vi "main.vi"() -> ()   [LabVIEW 2021]
panel:
  in  "VALHTSw":bool
  in  "Stop":bool
  in  "SPVALLT":u8 max=100
  in  "SPVALHT":u8 max=100
  out "DPTSYS":sgl format="%#_3g"
  out "DPTOT":sgl format="%#_2g"
  out "DPVALLT":sgl
  out "DPVALHT":sgl
  out "DPTEGLT":sgl
  out "DPTEGHT":sgl
  out "posVALLT":sgl(knob) scale=0.0..100.0
  out "posVALHT":sgl(knob) scale=0.0..100.0
  out "Boolean":bool
  # "%"
  # "%"
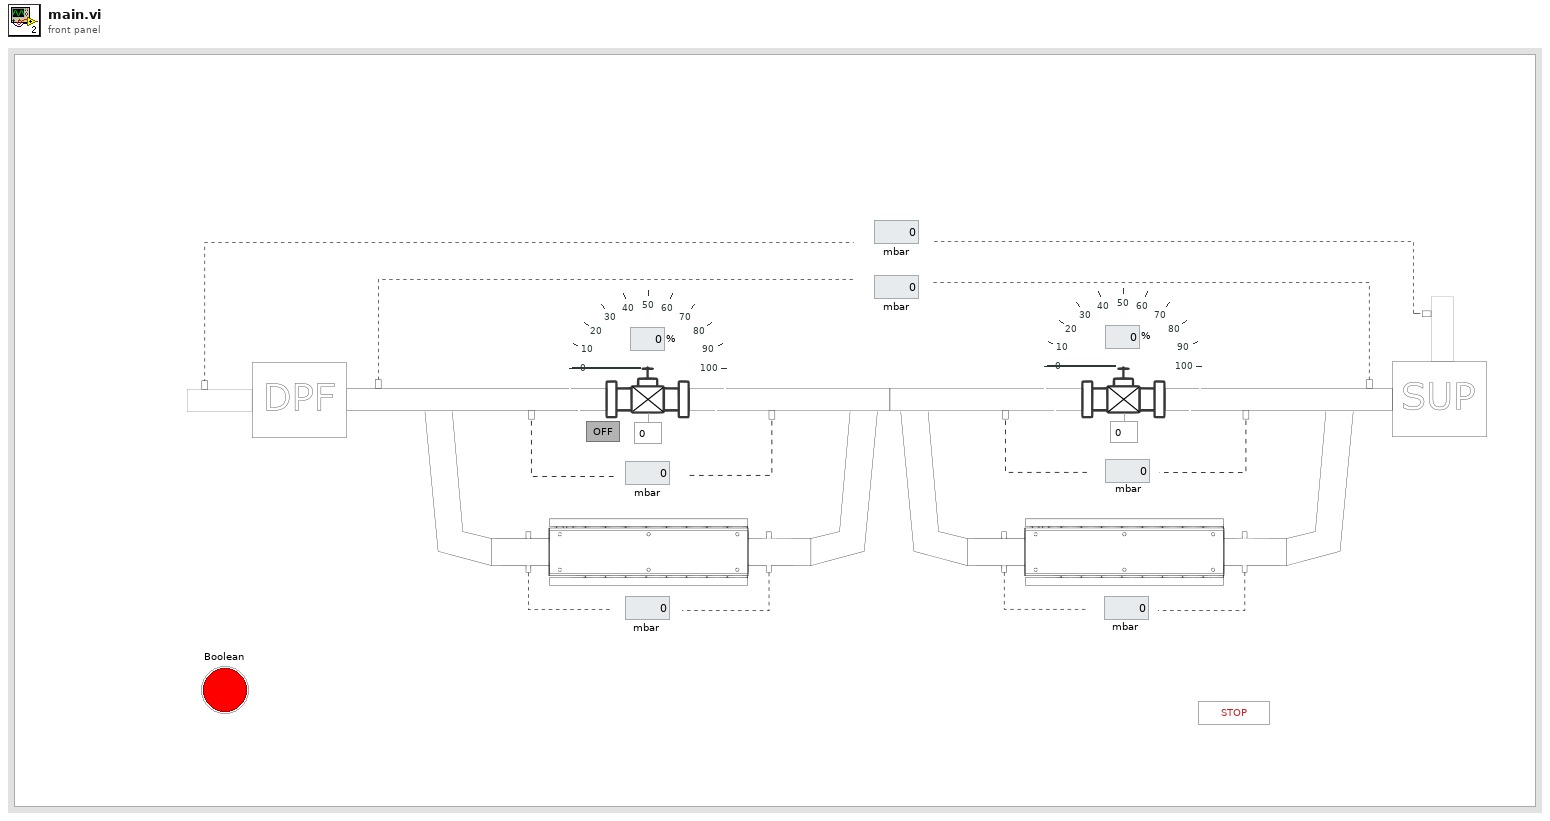
[diagram p1: front panel]
types:
  T1 = cluster{"ValvePos1":sgl, "ValvePos2":sgl, "PressureArray":sgl[], "TempArray2":sgl[], "TempArray1":sgl[]}[]
  T2 = enum16{"waiting", "connect to tcp server", "configuration", "data logging", "saving data and close connection"}
  T3 = enum16{"Disconnected", "Connecting", "Conected", "Sending"}
  T4 = cluster{"ValvePos1":i32, "ValvePos2":i32, "PressureArray":sgl[], "TempArray2":sgl[], "TempArray1":sgl[]}
  T5 = cluster{"ValvePos1":sgl, "ValvePos2":sgl, "PressureArray":sgl[], "TempArray2":sgl[], "TempArray1":sgl[]}
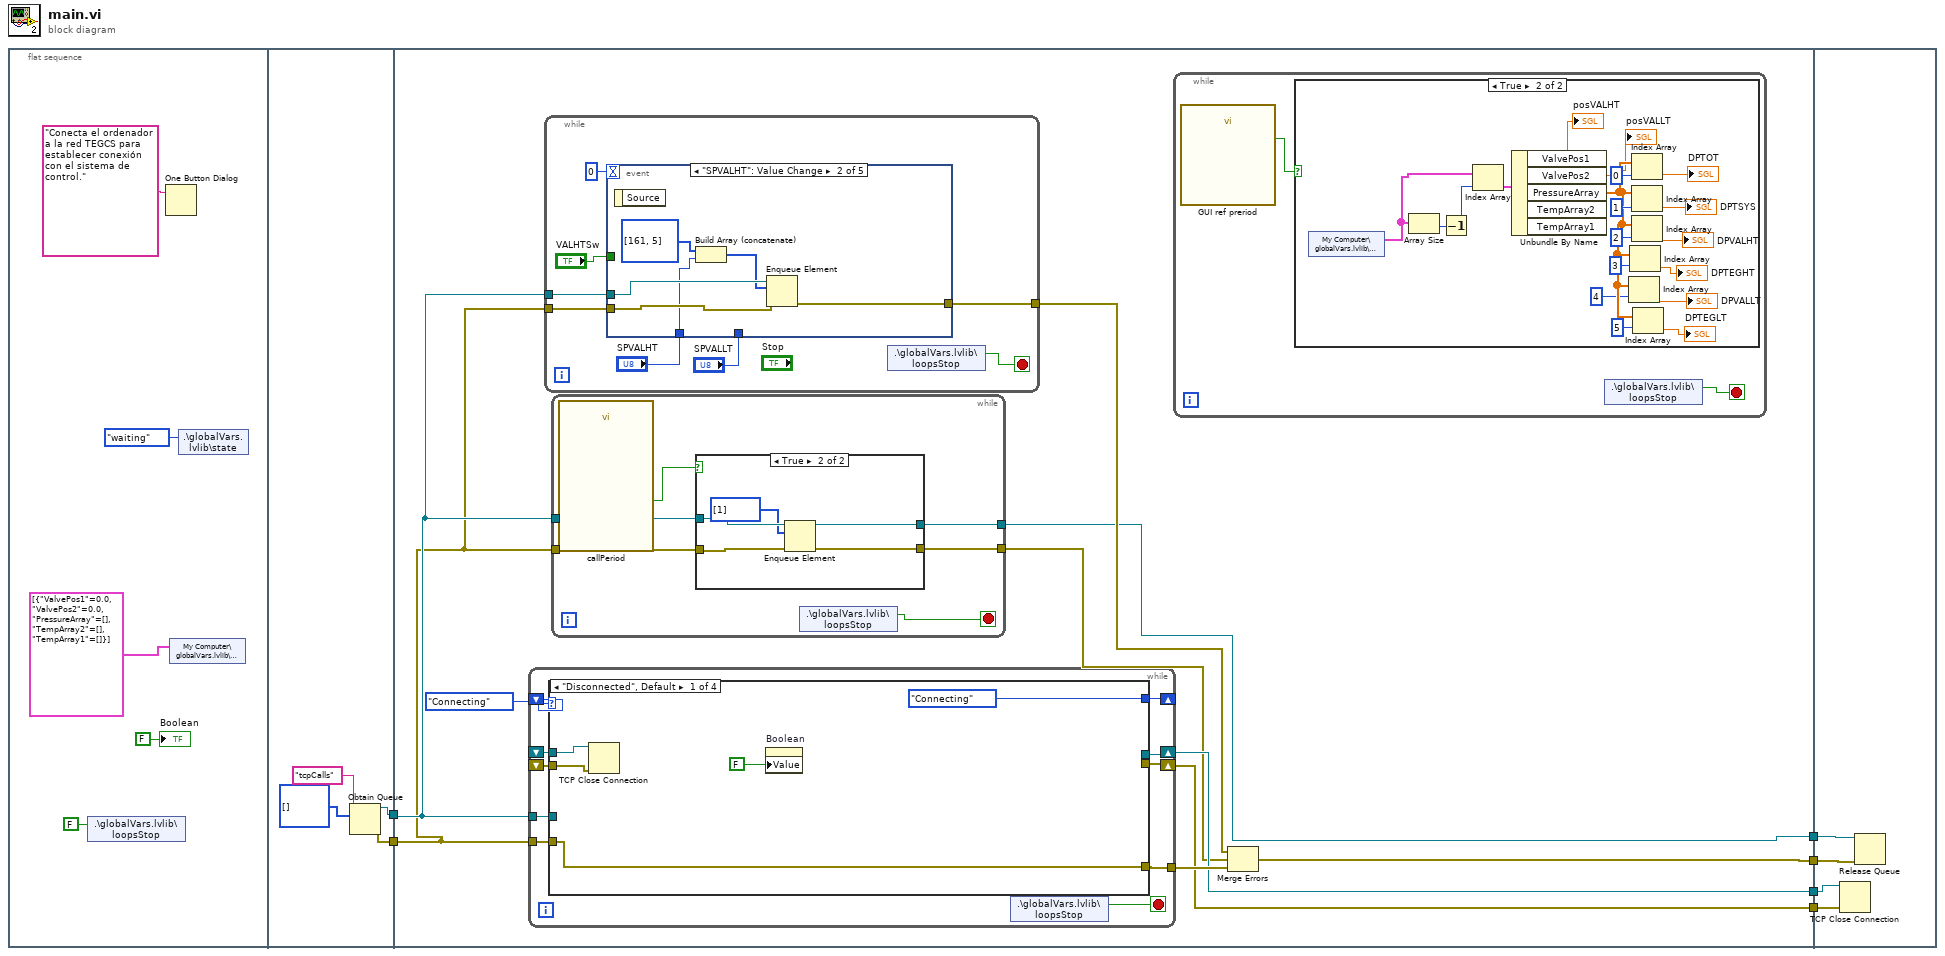
[diagram p0: block diagram]
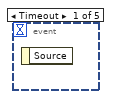
[diagram p2: hidden frame]
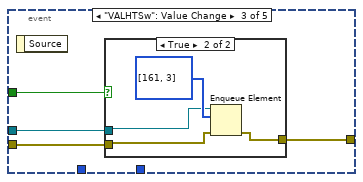
[diagram p3: hidden frame]
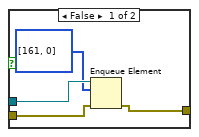
[diagram p4: hidden frame]
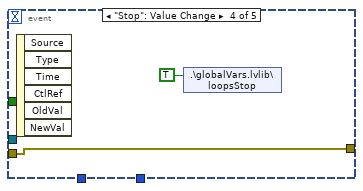
[diagram p5: hidden frame]
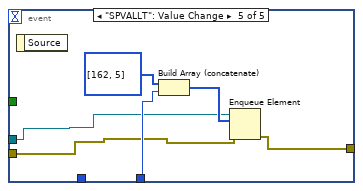
[diagram p6: hidden frame]
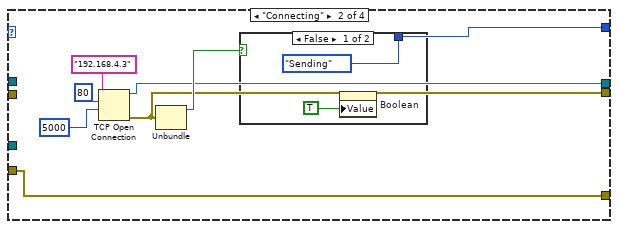
[diagram p9: hidden frame]
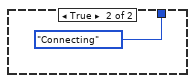
[diagram p10: hidden frame]
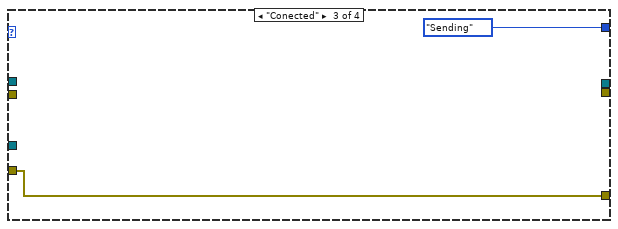
[diagram p11: hidden frame]
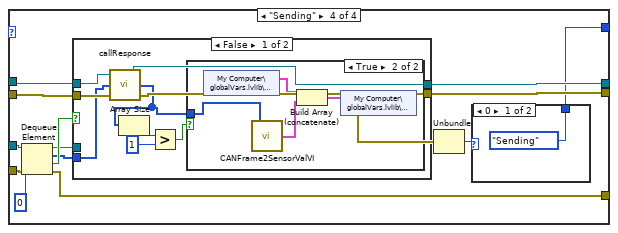
[diagram p12: hidden frame]
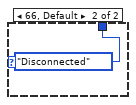
[diagram p13: hidden frame]
diagram:
  n1 = flat-sequence {
    tunnel: [w13] -> w6
    tunnel: [w12] -> w5
    tunnel: w6 -> [w23]
    tunnel: w5 -> [w24]
    tunnel: [w21] -> w4
    tunnel: [w16] -> w3
    tunnel: [w20] -> w2
    tunnel: [w19] -> w1
    tunnel: w4 -> [w155]
    tunnel: w3 -> [w154]
    tunnel: w2 -> [w153]
    tunnel: w1 -> [w152]
    frame #0 {
      n2 = shared-variable ".\\globalVars.lvlib\\loopsStop"(FALSE ("loopsStop")) -> ()  [unwired: 1 in, 1 out]
      n3 = One Button Dialog(message="Conecta el ordenador a la red TEGCS para establecer conexión con el sistema de control.") -> ()  [unwired: 1 in, 1 out]
      n4 = shared-variable "My Computer\\globalVars.lvlib\\sensD"(T1 [{"ValvePos1"=0.0, "ValvePos2"=0.0, "PressureArray"=[], "TempArray2"=[], "TempArray1"=[]}] ("sensD")) -> ()  [unwired: 1 in, 1 out]
      n5 = shared-variable ".\\globalVars.lvlib\\state"(T2."waiting" ("state")) -> ()  [unwired: 1 in, 1 out]
      "Boolean" <- FALSE ("Boolean")
    }
    frame #1 {
      n6 = Obtain Queue(name (unnamed)="tcpCalls", element data type=u8[] [] ("Array")) -> (queue out=w12:refnum<queue>, error out=w13:errorcluster)  [unwired: 3 in, 1 out]
    }
    frame #2 {
      n7 = while {
        shift-right: [w100] -> _
        shift-left: T3."Connecting" -> [w103]
        shift-right: [w102] -> w19
        shift-left: _ -> [w99]
        shift-right: [w101] -> w20
        shift-left: _ -> [w98]
        tunnel: w23 -> [w97]
        tunnel: w24 -> [w96]
        tunnel: [w94] -> w22
        stop <- w95 stop-if-true
        n8 = case shown="\"Disconnected\", Default" w103 {
          tunnel: [T3."Connecting" w113 T3."Sending" w125] -> w100
          tunnel: [_ w111 _ w128] -> w102
          tunnel: [_ w110 _ w127] -> w101
          tunnel: w99 -> [w108 _ _ w130]
          tunnel: w98 -> [w107 _ _ w129]
          tunnel: w97 -> [w104 w109 w120 w133]
          tunnel: w96 -> [_ _ _ w134]
          tunnel: [w104 w109 w120 w124] -> w94
          frame "Disconnected", Default {
            n9 = TCP Close Connection(connection ID=w108, error in (no error)=w107) -> ()  [unwired: 1 in, 2 out]
            n10 = property on="Boolean" class="Bool (strict)"("Value"=FALSE ("Boolean")) -> ()  [unwired: 2 in, 2 out]
          }
          frame "Connecting" {
            n11 = TCP Open Connection(address="192.168.4.3", remote port or service name=u16 80, timeout ms (60000)=5000) -> (connection ID=w111:refnum<k5>, error out=w110:errorcluster)  [unwired: 2 in]
            n12 = Unbundle(w110) -> ("status"=w112:bool)  [unwired: 2 out]
            n13 = case shown="False" w112 {
              tunnel: [T3."Sending" T3."Connecting"] -> w113
              frame False {
                n14 = property on="Boolean" class="Bool (strict)"("Value"=TRUE ("Boolean")) -> ()  [unwired: 2 in, 2 out]
              }
              frame True {
              }
            }
          }
          frame "Conected" {
          }
          frame "Sending" {
            n15 = Dequeue Element(queue=w134, timeout in ms (-1)=0, error in (no error)=w133) -> (queue out=w123:refnum<queue>, element=w122:u8[], timed out?=w131:bool, error out=w124:errorcluster)
            n16 = case shown="False" w131 {
              tunnel: w130 -> [w145 w150]
              tunnel: w129 -> [w144 w151]
              tunnel: [w143 w151] -> w127
              tunnel: [w142 w150] -> w128
              tunnel: w123 -> [_ _]
              tunnel: w122 -> [w141 _]
              frame False {
                n17 = call "callResponse.vi"("error in (no error)"=w144, "input"=w141, "TCP Network Connection in"=w145) -> ("error out"=w143:errorcluster, "unsigned byte array"=w137:u8[], "TCP Network Connection out"=w142:refnum<k5>)
                n18 = Array Size(array=w137) -> (size(s)=w140:i32)
                n19 = Greater?(x=w140, y=1) -> (0:w138:bool)
                n20 = case shown="True" w138 {
                  tunnel: w137 -> [_ w148]
                  frame False {
                  }
                  frame True {
                    n21 = shared-variable "My Computer\\globalVars.lvlib\\sensD"() -> (w146:T1)  [unwired: 1 in, 1 out]
                    n22 = call "CANFrame2SensorValVI.vi"("input"=w148) -> ("output data cluster"=w149:T4)
                    n23 = Build Array (concatenate)(w146, w149) -> (w147:T1)
                    n24 = shared-variable "My Computer\\globalVars.lvlib\\sensD"(w147) -> ()  [unwired: 1 in, 1 out]
                  }
                }
              }
              frame True {
              }
            }
            n25 = Unbundle(w127) -> ("code"=w126:i32)  [unwired: 2 out]
            n26 = case shown="0" w126 {
              tunnel: [T3."Sending" T3."Disconnected"] -> w125
              frame 0 {
              }
              frame 66, Default {
              }
            }
          }
        }
        n27 = shared-variable ".\\globalVars.lvlib\\loopsStop"() -> (w95:bool)  [unwired: 1 in, 1 out]
      }
      n28 = while {
        tunnel: w24 -> [w30]
        tunnel: w23 -> [w32]
        tunnel: [w27] -> w17
        stop <- w29 stop-if-true
        n29 = event shown="[1] \"SPVALHT\": Value Change" {
          selector: _ -> [_ _ _ _ _]
          dyn-events: _ -> [_ _ _ _ _]
          timeout: 0 -> [_ _ _ _ _]
          tunnel: w32 -> [_ w38 w43 w52 w56]
          tunnel: "SPVALHT" -> [_ w36 _ _ _]
          tunnel: w30 -> [_ w39 w42 _ w55]
          tunnel: "SPVALLT" -> [_ _ _ _ w57]
          tunnel: [_ w34 w40 w52 w54] -> w27
          tunnel: "VALHTSw" -> [_ _ w41 _ _]
          event Timeout {
            n30 = event-data() -> ()  [unwired: 1 in, 1 out]
          }
          event "SPVALHT": Value Change {
            n31 = event-data() -> ()  [unwired: 1 in, 1 out]
            n32 = Build Array (concatenate)(u8[] [161, 5] ("element"), w36) -> (w35:u8[])
            n33 = Enqueue Element(queue=w39, element=w35, error in (no error)=w38) -> (error out=w34:errorcluster)  [unwired: 1 in, 2 out]
          }
          event "VALHTSw": Value Change {
            n34 = event-data() -> ()  [unwired: 1 in, 1 out]
            n35 = case shown="True" w41 {
              tunnel: w43 -> [w47 w49]
              tunnel: w42 -> [w46 w50]
              tunnel: [w44 w48] -> w40
              frame False {
                n36 = Enqueue Element(queue=w46, element=u8[] [161, 0], error in (no error)=w47) -> (error out=w44:errorcluster)  [unwired: 1 in, 2 out]
              }
              frame True {
                n37 = Enqueue Element(queue=w50, element=u8[] [161, 3], error in (no error)=w49) -> (error out=w48:errorcluster)  [unwired: 1 in, 2 out]
              }
            }
          }
          event "Stop": Value Change {
            n38 = event-data() -> ()  [unwired: 1 in, 6 out]
            n39 = shared-variable ".\\globalVars.lvlib\\loopsStop"(TRUE ("loopsStop")) -> ()  [unwired: 1 in, 1 out]
          }
          event "SPVALLT": Value Change {
            n40 = event-data() -> ()  [unwired: 1 in, 1 out]
            n41 = Build Array (concatenate)(u8[] [162, 5] ("element"), w57) -> (w58:u8[])
            n42 = Enqueue Element(queue=w55, element=w58, error in (no error)=w56) -> (error out=w54:errorcluster)  [unwired: 1 in, 2 out]
          }
        }
        n43 = shared-variable ".\\globalVars.lvlib\\loopsStop"() -> (w29:bool)  [unwired: 1 in, 1 out]
      }
      n44 = while {
        tunnel: w24 -> [w84]
        tunnel: w23 -> [w85]
        tunnel: [w83] -> w18
        tunnel: [w82] -> w16
        stop <- w81 stop-if-true
        n45 = call "callPeriod"() -> ("Time has Elapsed"=w86:bool)  [unwired: 12 in, 7 out]
        n46 = case shown="True" w86 {
          tunnel: w85 -> [w88 w92]
          tunnel: w84 -> [w87 w93]
          tunnel: [w88 w90] -> w83
          tunnel: [w87 w89] -> w82
          frame False {
          }
          frame True {
            n47 = Enqueue Element(queue=w93, element=u8[] [1], error in (no error)=w92) -> (queue out=w89:refnum<queue>, error out=w90:errorcluster)  [unwired: 1 in, 1 out]
          }
        }
        n48 = shared-variable ".\\globalVars.lvlib\\loopsStop"() -> (w81:bool)  [unwired: 1 in, 1 out]
      }
      n49 = while {
        stop <- w61 stop-if-true
        n50 = call "GUI ref preriod"() -> ("Time has Elapsed"=w60:bool)  [unwired: 12 in, 7 out]
        n51 = case shown="True" w60 {
          frame False {
          }
          frame True {
            n52 = shared-variable "My Computer\\globalVars.lvlib\\sensD"() -> (w62:T1)  [unwired: 1 in, 1 out]
            n53 = Array Size(array=w62) -> (size(s)=w80:i32)
            n54 = Decrement(x=w80) -> (x-1=w79:i32)
            n55 = Index Array(array=w62, index=w79) -> (element=w78:T5)
            n56 = Unbundle By Name(w78) -> ("ValvePos1"=→"posVALHT":sgl, "ValvePos2"=→"posVALLT":sgl, "PressureArray"=w67:sgl[])  [unwired: 2 out]
            n57 = Index Array(array=w67, index=4) -> (element=→"DPVALLT":sgl)
            n58 = Index Array(array=w67, index=3) -> (element=→"DPTEGHT":sgl)
            n59 = Index Array(array=w67, index=0) -> (element=→"DPTOT":sgl)
            n60 = Index Array(array=w67, index=1) -> (element=→"DPTSYS":sgl)
            n61 = Index Array(array=w67, index=2) -> (element=→"DPVALHT":sgl)
            n62 = Index Array(array=w67, index=5) -> (element=→"DPTEGLT":sgl)
          }
        }
        n63 = shared-variable ".\\globalVars.lvlib\\loopsStop"() -> (w61:bool)  [unwired: 1 in, 1 out]
      }
      n64 = Merge Errors(w17, w18, w22) -> (w21:errorcluster)
    }
    frame #3 {
      n65 = TCP Close Connection(connection ID=w152, error in (no error)=w153) -> ()  [unwired: 1 in, 2 out]
      n66 = Release Queue(queue=w154, error in (no error)=w155) -> ()  [unwired: 1 in, 3 out]
    }
  }
